vi "SCLN_InitClient.vi"(1 "error in (no error)":errorcluster, 3 "Config File Name":path, 4 "Server Name":string) -> (0 "error out":errorcluster)   [LabVIEW 2015]
uses:
  SCLN_RW_Select.ctl
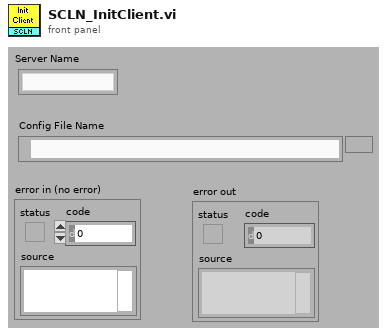
[diagram p1: front panel]
types:
  T1 = typedef "SCLN_InfoClusterConfig.ctl" = cluster{"Section Name":string, "IP_Server":string, "IP_Client":string, "IP_Port":string}
  T2 = typedef "SCLN_RW_Select.ctl" = enum16{"Read", "Write"}
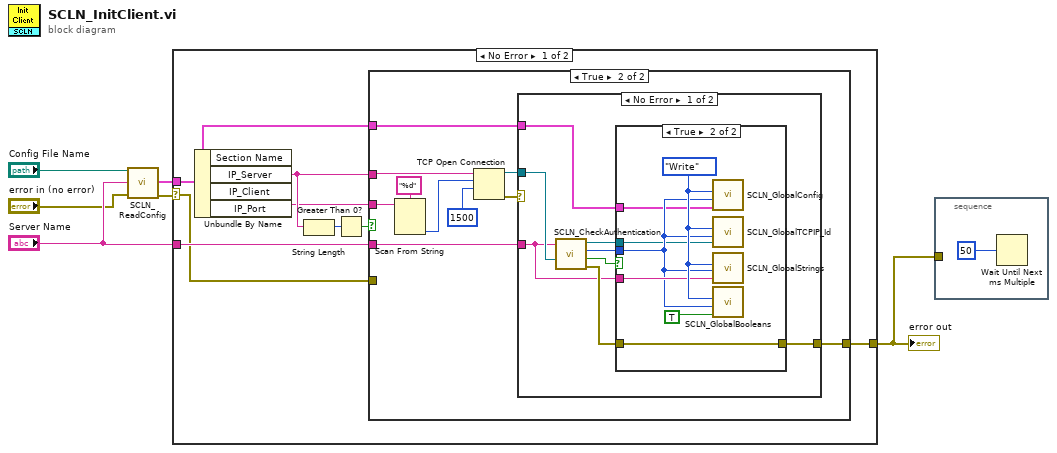
[diagram p0: block diagram]
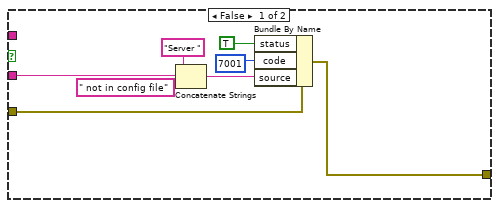
[diagram p2: hidden frame]
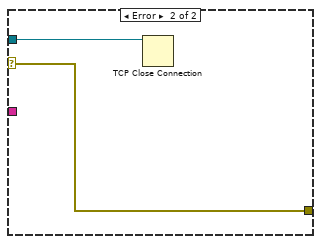
[diagram p4: hidden frame]
diagram:
  n1 = call "SCLN_ReadConfig.vi"("File Path"="Config File Name", "Section Name"="Server Name", "error in (no error)"="error in (no error)") -> ("IP Info Connection"=w5:T1, "error out"=w4:errorcluster)  [unwired: 11 in]
  n2 = case shown="No Error" w4 {
    selector: w4 -> [w7 w51]
    tunnel: w5 -> [w10 _]
    tunnel: [w9 w51] -> w1
    tunnel: "Server Name" -> [w8 _]
    frame No Error {
      n3 = Unbundle By Name(w10) -> ("IP_Server"=w12:string, "IP_Port"=w11:string)  [unwired: 2 out]
      n4 = String Length(string=w12) -> (length=w14:i32)
      n5 = Greater Than 0?(x=w14) -> (x > 0?=w13:bool)
      n6 = case shown="True" w13 {
        tunnel: w12 -> [_ w30]
        tunnel: w11 -> [_ w31]
        tunnel: w10 -> [_ w27]
        tunnel: [w17 w23] -> w9
        tunnel: w8 -> [w16 w24]
        tunnel: w7 -> [w15 _]
        frame False {
          n7 = Concatenate Strings("Server ", w16, " not in config file") -> (w18:string)
          n8 = Bundle By Name(cluster=w15, "status"=TRUE, "code"=7001, "source"=w18) -> (w17:errorcluster)
        }
        frame True {
          n9 = Scan From String(format string="%d", input string=w31) -> (output 1=w29:i32)  [unwired: 3 in, 3 out]
          n10 = TCP Open Connection(address=w30, remote port or service name=w29, timeout ms (60000)=1500) -> (connection ID=w26:refnum<k5>, error out=w25:errorcluster)  [unwired: 2 in]
          n11 = case shown="No Error" w25 {
            selector: w25 -> [_ w50]
            tunnel: w27 -> [w34 _]
            tunnel: w26 -> [w40 w49]
            tunnel: w24 -> [w35 _]
            tunnel: [w33 w50] -> w23
            frame No Error {
              n12 = call "SCLN_CheckAuthentication.vi"("Server Name"=w35, "TCP IN"=w40) -> ("TCP OUT"=w36:refnum<k5>, "Client Index"=w37:i32, "Authentic"=w39:bool, "error out"=w38:errorcluster)
              n13 = case shown="True" w39 {
                tunnel: w38 -> [w41 w42]
                tunnel: w37 -> [_ w45]
                tunnel: w36 -> [_ w44]
                tunnel: w35 -> [_ w46]
                tunnel: w34 -> [_ w43]
                tunnel: [w41 w42] -> w33
                frame False {
                }
                frame True {
                  w48 = SCLN_RW_Select."Write" ("GBL_RW")
                  n14 = call "SCLN_GlobalConfig.vi"("Write Value"=w43, "Element"=w45, "Operation"=w48) -> ()  [unwired: 1 in, 2 out]
                  n15 = call "SCLN_GlobalTCPIP_Id.vi"("TCPIP_Id Write"=w44, "Element"=w45, "Operation"=w48) -> ()  [unwired: 1 in, 2 out]
                  n16 = call "SCLN_GlobalStrings.vi"("Write Value"=w46, "Element"=w45, "Operation"=w48) -> ()  [unwired: 1 in, 2 out]
                  n17 = call "SCLN_GlobalBooleans.vi"("Write Value"=TRUE, "Element"=w45, "Operation"=w48) -> ()  [unwired: 1 in, 2 out]
                }
              }
            }
            frame Error {
              n18 = TCP Close Connection(connection ID=w49) -> ()  [unwired: 2 in, 2 out]
            }
          }
        }
      }
    }
    frame Error {
    }
  }
  "error out" <- w1
  n19 = stacked-sequence {
    tunnel: w1 -> [_]
    frame #0 {
      n20 = Wait Until Next ms Multiple(millisecond multiple=50) -> ()  [unwired: 1 out]
    }
  }
